vi "Initialize Device Core.vi"(8 "error in (no error)":errorcluster, 9 "Reset (F)":bool, 10 "Resource Name":string, 11 "CS++Scope in":refnum<class "CS++Scope.lvclass">) -> (0 "error out":errorcluster, 3 "CS++Scope out":refnum<class "CS++Scope.lvclass">)   [LabVIEW 2013, in "CS++Scope.lvlib" / "CS++Scope.lvclass"]
doc: "Initialize device driver."
uses:
  CS++Scope.lvclass
  CSPP_Core/Actors/CS++DeviceActor/CS++DeviceActor.lvclass
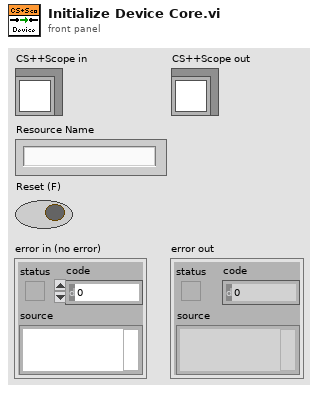
[diagram p1: front panel]
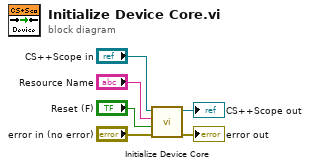
[diagram p0: block diagram]
diagram:
  n1 = call-parent "Initialize Device Core.vi"("error in (no error)"="error in (no error)", "Reset (F)"="Reset (F)", "Resource Name"="Resource Name", "CS++DeviceActor in"="CS++Scope in") -> ("error out"=→"error out":errorcluster, "CS++DeviceActor out"=→"CS++Scope out":refnum<class "CS++Scope.lvclass">)  [unwired: 6 in]
